vi "Swerve Module (Metric).vi"(0 "Y":dbl, 1 "X":dbl, 2 "Gyroscope":dbl, 3 "Rotation":dbl, 4 "alpha":dbl=50.64 format="%#_13g", 5 "error in":errorcluster, 7 "Steering Motor type":i32(ring) items=["Talon FX", "SPARK MAX", "Talon SRX"], 9 "Drive Motor type":i32(ring) items=["Talon FX", "SPARK MAX", "Talon SRX"], 11 "ticks per rev":dbl=2048.0 format="%#_13g", 13 "Gear Ratio":dbl=15.4286 format="%#_13g") -> (14 "Angle Out":dbl[](array[numeric]), 16 "Steering Postion Control":dbl[](array[numeric]), 18 "Drive Power":dbl[](array[numeric]), 19 "error out":errorcluster)   [LabVIEW 2020]
uses:
  <vilib>/Analysis/coordinate.llb/Angle Units.ctl
  <vilib>/Analysis/coordinate.llb/Angle Range (Degree).ctl
  <vilib>/Rock Robotics/WPI/ThirdParty/Phoenix-LabVIEW/Motor Controller/Controls/CTRE_Phoenix_MotorControl_TalonFXInvertType.ctl
  <vilib>/Analysis/coordinate.llb/Wrap Angle (scalar).vi
  <vilib>/Rock Robotics/WPI/ThirdParty/JAS_Junk/TrajLib/Conv_Deg_Radians.vi
  <vilib>/Rock Robotics/WPI/ThirdParty/JAS_Junk/TrajLib/Rotation2d_CreateAngle.vi
  <vilib>/Rock Robotics/WPI/ThirdParty/JAS_Junk/TrajLib/Util_CalcDist.vi
  <vilib>/Rock Robotics/WPI/ThirdParty/JAS_Junk/TrajLib/Rotation2d_UnaryMinus.vi
  <vilib>/Rock Robotics/WPI/Utilities/WPI_GetSetVariantRefNum.vi
  <vilib>/Rock Robotics/WPI/ThirdParty/Phoenix-LabVIEW/CANCoder/Get/CTRE_Phoenix_CANcoder_GetSensorData.vi
  <vilib>/Rock Robotics/WPI/ThirdParty/Phoenix-LabVIEW/Motor Controller/Get/CTRE_Phoenix_MotorController_GetSelectedSensorData.vi
  <vilib>/Rock Robotics/WPI/ThirdParty/JAS_Junk/TrajLib/Trajectory_Library.lvlib
  <vilib>/Analysis/NI_AAL_Angle.lvlib
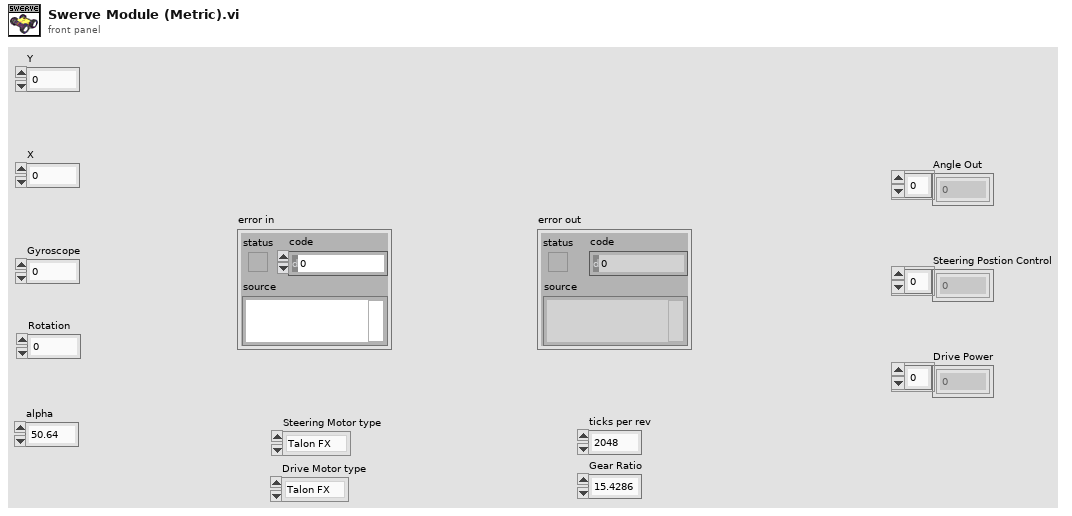
[diagram p1: front panel]
types:
  T1 = typedef "NI_AAL_Angle.lvlib/Angle Range (Degree).ctl" = u16
  T2 = typedef "NI_AAL_Angle.lvlib/Angle Units.ctl" = i32
  T3 = typedef "CTRE_Phoenix_CANcoder_DeviceRef.ctl" = cluster{"DeviceStatus":errorcluster, "Device Number":u8, "Handle":u64, "UsageFrame":u32, "Library Path":path}
  T4 = typedef "WPI_MotorControlDeviceRef.ctl" = cluster{"DeviceStatus":errorcluster, "Type":T5, "PWM":cluster{"PWM Channel":T6, "DeadBand":T7}, "CAN":cluster{"Device Number":u8, "SetOutput VI Ref":variant, "GetOutput VI Ref":variant, "Enable VI Ref":variant, "Disable VI Ref":variant, "Data":variant}, "Invert":bool, "DIO PWM":cluster{"PWM \"Enable\" Channel":T6, "DIOChannel":T8, "PWM Rate":dbl}}
  T5 = typedef "WPI_MotorControlType.ctl" = enum16{"PWM", "CAN", "DIO PWM"}
  T6 = typedef "FPGA_DIOPWMChannel.ctl" = enum8{"PWM 0", "PWM 1", "PWM 2", "PWM 3", "PWM 4", "PWM 5", "PWM 6", "PWM 7", "PWM 8", "PWM 9", "PWM MXP 0", "PWM MXP 1", "PWM MXP 2", "PWM MXP 3", "PWM MXP 4", "PWM MXP 5", "PWM MXP 6", "PWM MXP 7", "PWM MXP 8", "PWM MXP 9", "Invalid"}
  T7 = typedef "WPI_PWMDeadband.ctl" = cluster{"Name":string, "maxPositivePwm":i32, "minPositivePwm":i32, "centerPwm":i32, "maxNegativePwm":i32, "minNegativePwm":i32, "angularRange":u16}
  T8 = typedef "FPGA_DIOChannel.ctl" = enum8{"DIO 0", "DIO 1", "DIO 2", "DIO 3", "DIO 4", "DIO 5", "DIO 6", "DIO 7", "DIO 8", "DIO 9", "DIO MXP 0", "DIO MXP 1", "DIO MXP 2", "DIO MXP 3", "DIO MXP 4", "DIO MXP 5", "DIO MXP 6", "DIO MXP 7", "DIO MXP 8", "DIO MXP 9", "DIO MXP 10", "DIO MXP 11", "DIO MXP 12", "DIO MXP 13", "DIO MXP 14", "DIO MXP 15", "SPI Port CS1", "SPI Port CS2", "SPI Port CS3", "SPI Port MISO", "SPI Port MOSI", "Invalid"}
  T9 = typedef "Trajectory_Library.lvlib/ROTATION2D.ctl" = cluster{"VALUE":dbl, "COS":dbl, "SIN":dbl}
  T10 = typedef "WPI_JoystickDevRef.ctl" = cluster{"Device":T11}
  T11 = typedef "WPI_JoystickDeviceEnum.ctl" = enum16{"USB 0", "USB 1", "USB 2", "USB 3", "USB 4", "USB 5"}
  T12 = typedef "CTRE_Phoenix_MotorControl_TalonFXInvertType.ctl" = enum16{"Counter-Clockwise", "Clockwise"}
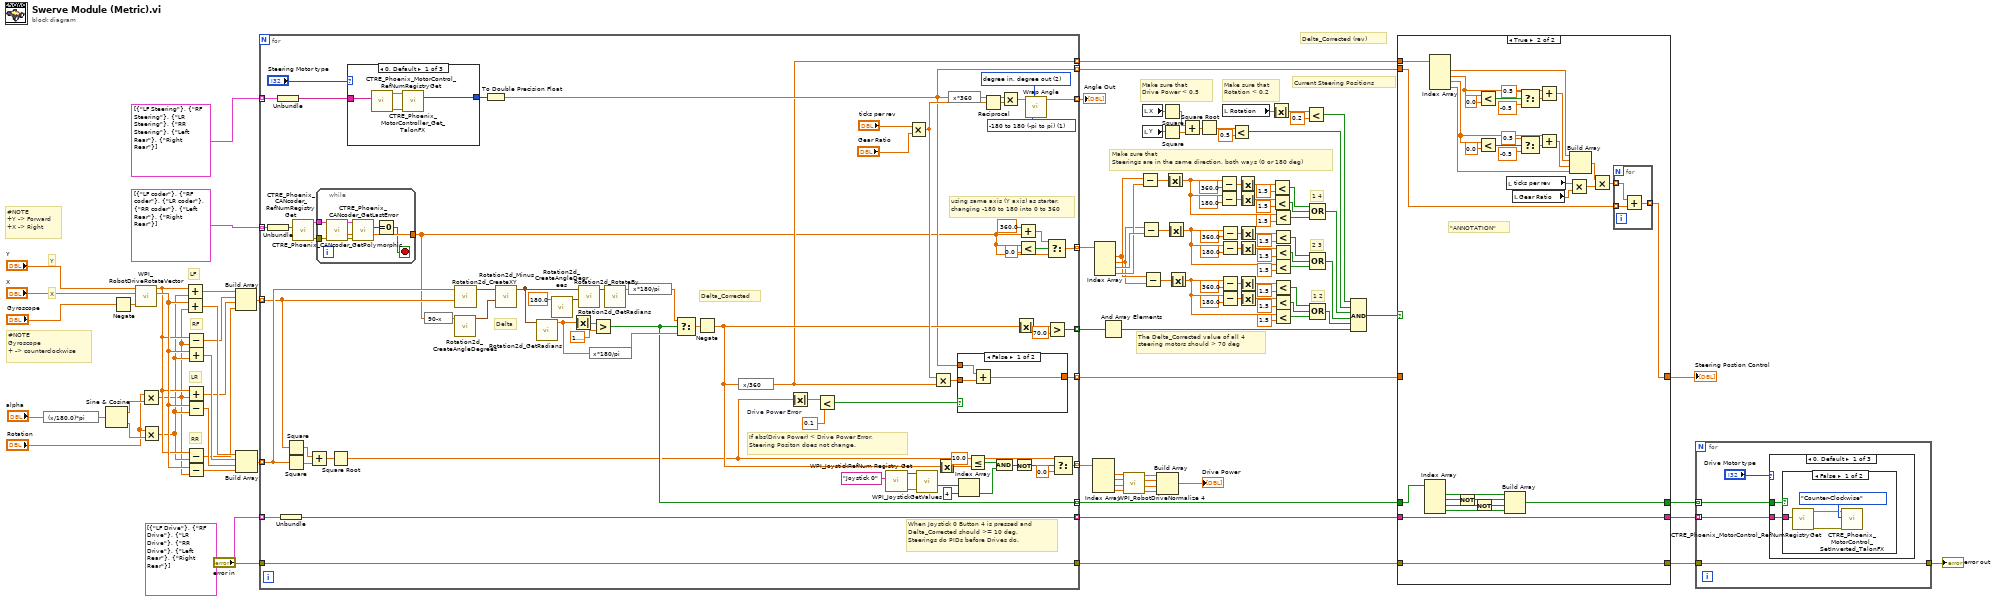
[diagram p0: block diagram]
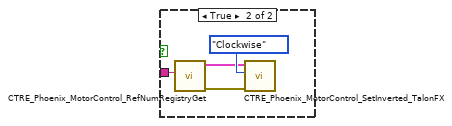
[diagram p3: hidden frame]
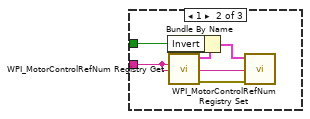
[diagram p4: hidden frame]
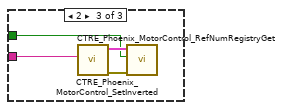
[diagram p5: hidden frame]
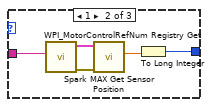
[diagram p6: hidden frame]
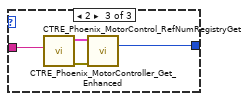
[diagram p7: hidden frame]
diagram:
  # "#NOTE\nGyroscope\n+ -> counterclockwise"
  # "#NOTE\n+Y -> Forward\n+X -> Right"
  # "Current Steering Positions"
  # "Delta_Corrected (rev)"
  # "Make sure that\nRotation < 0.2"
  # "Make sure that\nDrive Power < 0.5"
  # "The Delta_Corrected value of all 4 steering motors should > 70 deg"
  # "Make sure that\nSteerings are in the same direction, both ways (0 or 180 deg)"
  # "1 4"
  # "1 2"
  # "2 3"
  # "RR"
  # "LR"
  # "RF"
  # "LF"
  # "X"
  # "Y"
  n1 = expression code="(x/180.0)*pi" ("degrees to radians")("alpha") -> (w83:dbl)
  n2 = Sine & Cosine(0:w83) -> (1:w85:dbl, 2:w84:dbl)
  n3 = Negate(x="Gyroscope") -> (-x=w2:dbl)
  n4 = call <vilib>:"WPI_RobotDriveRotateVector.vi"("Angle"=w2, "X"="X", "Y"="Y") -> ("X'"=w90:dbl, "Y'"=w89:dbl)  [unwired: 7 out]
  n5 = Multiply(x="Rotation", y=w85) -> (x*y=w87:dbl)
  n6 = Multiply(x="Rotation", y=w84) -> (x*y=w88:dbl)
  n7 = Add(x=w89, y=w88) -> (x+y=w92:dbl)
  n8 = Add(x=w90, y=w87) -> (x+y=w96:dbl)
  n9 = Subtract(x=w89, y=w87) -> (x-y=w93:dbl)
  n10 = Add(x=w90, y=w88) -> (x+y=w97:dbl)
  n11 = Add(x=w89, y=w87) -> (x+y=w94:dbl)
  n12 = Subtract(x=w90, y=w88) -> (x-y=w98:dbl)
  n13 = Subtract(x=w89, y=w88) -> (x-y=w95:dbl)
  n14 = Subtract(x=w90, y=w87) -> (x-y=w99:dbl)
  n15 = Build Array(w92, w93, w94, w95) -> (w100:dbl[])
  n16 = Build Array(w96, w97, w98, w99) -> (w101:dbl[])
  n17 = for {
    tunnel: w100 -> [w147] mode=indexing
    tunnel: w101 -> [w148] mode=indexing
    tunnel: [w129] -> w108 mode=indexing
    tunnel: cluster{string}[] [{"LF Steering"}, {"RF Steering"}, {"LR Steering"}, {"RR Steering"}, {"Left Rear"}, {"Right Rear"}] ("Steering ref") -> [w182] mode=indexing
    tunnel: cluster{string}[] [{"LF coder"}, {"RF coder"}, {"LR coder"}, {"RR coder"}, {"Left Rear"}, {"Right Rear"}] ("CANcoder ref") -> [w178] mode=indexing
    tunnel: cluster{string}[] [{"LF Drive"}, {"RF Drive"}, {"LR Drive"}, {"RR Drive"}, {"Left Rear"}, {"Right Rear"}] ("Drive ref") -> [w173] mode=indexing
    tunnel: [w172] -> w77 mode=indexing
    tunnel: [w133] -> w48 mode=indexing
    tunnel: "error in" -> [w163]
    tunnel: [w163] -> w75
    tunnel: [w146] -> w81 mode=indexing
    tunnel: [w145] -> w79 mode=indexing
    tunnel: [w142] -> w49 mode=indexing
    tunnel: [w137] -> w50 mode=indexing
    tunnel: [w117] -> w6 mode=indexing
    tunnel: [w116] -> w5 mode=indexing
    w136 = T1 1 items=["none", "-180 to 180 (-pi to pi)", "0 to 360 (0 to 2pi)"] ("angle range")
    w135 = T2 2 items=["radian in, radian out", "radian in, degree out", "degree in, degree out", "degree in, radian out"] ("angle units")
    w175 = 0.1  # Drive Power Error
    # "When Joystick 0 Button 4 is pressed and Delta_Corrected should >= 10 deg,\nSteerings do PIDs before Drives do."
    # "Delta_Corrected"
    # "using same axis (Y axis) as starter,\nchanging -180 to 180 into 0 to 360"
    # "If abs(Drive Power) < Drive Power Error,\nSteering Positon does not change."
    # "Delta"
    n18 = Unbundle(w178) -> (w177:string)
    n19 = Unbundle(w182) -> (w181:string)
    n20 = Unbundle(w173) -> (w146:string)
    n21 = Square(x=w147) -> (x^2=w183:dbl)
    n22 = Square(x=w148) -> (x^2=w184:dbl)
    n23 = call <vilib>:"CTRE_Phoenix_CANcoder_RefNumRegistryGet.vi"("refnum name"=w177) -> ("error out"=w180:errorcluster, "CTRE_CANcoder_DeviceRef"=w179:T3)  [unwired: 9 in]
    n24 = Add(x=w183, y=w184) -> (x+y=w185:dbl)
    n25 = while {
      tunnel: w180 -> [w192]
      tunnel: w179 -> [w191]
      tunnel: [w187] -> w115
      stop <- w186 stop-if-true
      n26 = call-poly <vilib>:"CTRE_Phoenix_CANcoder_GetPolymorphic.vi"("CTRE_CANcoder_DeviceRef"=w191, "error in"=w192) -> ("CTRE_CANcoder_DeviceRef"=w190:T3, "Absolute Position"=w187:dbl, "error out"=w189:errorcluster)  [unwired: 9 in, 2 out]
      n27 = call <vilib>:"CTRE_Phoenix_CANcoder_GetLastError.vi"("error in"=w189, "CTRE_CANcoder_DeviceRef"=w190) -> ("Last Error Code"=w188:i8)  [unwired: 7 in, 2 out]
      n28 = Equal To 0?(x=w188) -> (x = 0?=w186:bool)
    }
    n29 = Square Root(x=w185) -> (sqrt(x)=w130:dbl)
    n30 = case shown="0, Default" "Steering Motor type" {
      tunnel: w181 -> [w194 w201 w203]
      tunnel: [w193 w197 w202] -> w176
      frame 0, Default {
        n31 = call <vilib>:"CTRE_Phoenix_MotorControl_RefNumRegistryGet.vi"("refnum name"=w194) -> ("error out"=w196:errorcluster, "PhoenixMotorControlDevRef"=w195:T4)  [unwired: 9 in]
        n32 = call-poly <vilib>:"CTRE_Phoenix_MotorController_Get_TalonFX.vi"("PhoenixMotorControlDevRef"=w195, "error in"=w196) -> ("Position (Raw Sensor Units)"=w193:i32)  [unwired: 10 in, 3 out]
      }
      frame 1 {
        n33 = call <vilib>:"WPI_MotorControlRefNum Registry Get.vi"("refnum name"=w201) -> ("error out"=w200:errorcluster, "MotorControlDevRef"=w199:T4)  [unwired: 9 in]
        n34 = call <vilib>:"Spark MAX Get Sensor Position.vi"("error in (no error)"=w200, "MotorControlDevRef in"=w199) -> ("Sensor Position"=w198:dbl)  [unwired: 6 in, 3 out]
        n35 = To Long Integer(number=w198) -> (32bit integer=w197:i32)
      }
      frame 2 {
        n36 = call <vilib>:"CTRE_Phoenix_MotorControl_RefNumRegistryGet.vi"("refnum name"=w203) -> ("error out"=w204:errorcluster, "PhoenixMotorControlDevRef"=w205:T4)  [unwired: 9 in]
        n37 = call-poly <vilib>:"CTRE_Phoenix_MotorController_Get_Enhanced.vi"("PhoenixMotorControlDevRef"=w205, "error in"=w204) -> ("Position (Raw Sensor Units)"=w202:i32)  [unwired: 10 in, 3 out]
      }
    }
    n38 = expression code="90-x"(w115) -> (w160:dbl)
    n39 = call <vilib>:"Rotation2d_CreateAngleDegrees.vi"("Angle_Degrees"=w160) -> ("ROTATION"=w159:T9)  [unwired: 10 in]
    n40 = call <vilib>:"Rotation2d_CreateXY.vi"("Y or sine"=w147, "X or  cosine"=w148) -> ("ROTATION"=w158:T9)  [unwired: 9 in]
    n41 = To Double Precision Float(number=w176) -> (double precision float=w117:dbl)
    n42 = call <vilib>:"Rotation2d_Minus.vi"("other ROTATION"=w159, "in ROTATION"=w158) -> ("out ROTATION"=w154:T9)  [unwired: 9 in]
    n43 = call <vilib>:"Rotation2d_GetRadians.vi"("in ROTATION"=w154) -> ("AngleRadians"=w157:dbl)  [unwired: 10 in]
    n44 = call <vilib>:"Rotation2d_CreateAngleDegrees.vi"("Angle_Degrees"=180.0) -> ("ROTATION"=w156:T9)  [unwired: 10 in]
    n45 = Absolute Value(x=w157) -> (abs(x)=w161:dbl)
    n46 = call <vilib>:"Rotation2d_RotateBy.vi"("other Rotation"=w156, "in ROTATION"=w154) -> ("out ROTATION"=w153:T9)  [unwired: 9 in]
    n47 = expression code="x*180/pi"(w157) -> (w150:dbl)
    n48 = Greater?(x=w161, y=1.5707963267948966) -> (0:w145:bool)
    n49 = call <vilib>:"Rotation2d_GetRadians.vi"("in ROTATION"=w153) -> ("AngleRadians"=w152:dbl)  [unwired: 10 in]
    n50 = expression code="x*180/pi"(w152) -> (w151:dbl)
    n51 = Select(t=w151, s=w145, f=w150) -> (s? t:f=w149:dbl)
    n52 = Negate(x=w149) -> (-x=w132:dbl)
    n53 = expression code="x/360"(w132) -> (w116:dbl)
    n54 = Absolute Value(x=w130) -> (abs(x)=w174:dbl)
    n55 = Less?(x=w174, y=w175) -> (x < y?=w171:bool)
    n56 = call <vilib>:"WPI_JoystickRefNum Registry Get.vi"("refnum name"="Joystick 0") -> ("error out"=w122:errorcluster, "JoystickDevRef"=w123:T10)  [unwired: 1 in, 8 out]
    n57 = Multiply(x="ticks per rev", y="Gear Ratio") -> (x*y=w164:dbl)
    n58 = call <vilib>:"WPI_JoystickGetValues.vi"("error in (no error)"=w122, "JoystickDevRef"=w123) -> ("Buttons"=w124:bool[])  [unwired: 5 in, 4 out]
    n59 = Multiply(x=w164, y=w116) -> (x*y=w165:dbl)
    n60 = Absolute Value(x=w132) -> (abs(x)=w126:dbl)
    n61 = expression code="x*360"(w117) -> (w166:dbl)
    n62 = case shown="False" w171 {
      tunnel: w165 -> [w208 _]
      tunnel: [w207 w209] -> w172
      tunnel: w117 -> [w206 w209]
      frame False {
        n63 = Add(x=w206, y=w208) -> (x+y=w207:dbl)
      }
      frame True {
      }
    }
    n64 = Index Array(array=w124, index=4) -> (element=w119:bool)
    n65 = Less Or Equal?(x=10.0, y=w126) -> (x <= y?=w131:bool)
    n66 = Reciprocal(x=w164) -> (1/x=w167:dbl)
    n67 = And(x=w131, y=w119) -> (x .and. y?=w128:bool)
    n68 = Multiply(x=w166, y=w167) -> (x*y=w134:dbl)
    n69 = Not(x=w128) -> (.not. x?=w127:bool)
    n70 = Absolute Value(x=w132) -> (abs(x)=w144:dbl)
    n71 = Add(x=360.0, y=w115) -> (x+y=w140:dbl)
    n72 = Less?(x=w115, y=0.0) -> (x < y?=w139:bool)
    n73 = call-poly <vilib>:"Wrap Angle.vi"("angle units"=w135, "angle range"=w136, "angle in"=w134) -> ("angle out"=w133:dbl)  [unwired: 7 in, 1 out]
    n74 = Select(t=w140, s=w139, f=w115) -> (s? t:f=w137:dbl)
    n75 = Greater?(x=w144, y=70.0) -> (0:w142:bool)
    n76 = Select(t=w130, s=w127, f=0.0) -> (s? t:f=w129:dbl)
  }
  "Angle Out" <- w48
  n77 = Index Array(array=w108) -> (element #1=w102:dbl, element #2=w103:dbl, element #3=w104:dbl, element #4=w105:dbl)  [unwired: 4 in]
  n78 = Index Array(array=w50) -> (element #1=w65:dbl, element #2=w64:dbl, element #3=w72:dbl, element #4=w69:dbl)  [unwired: 4 in]
  n79 = And Array Elements(Boolean array=w49) -> (logical AND=w23:bool)
  n80 = call <vilib>:"WPI_RobotDriveNormalize 4.vi"("D"=w105, "C"=w104, "B"=w103, "A"=w102) -> ("D'"=w111:dbl, "C'"=w112:dbl, "B'"=w113:dbl, "A'"=w114:dbl)
  n81 = Subtract(x=w65, y=w69) -> (x-y=w71:dbl)
  n82 = Subtract(x=w64, y=w72) -> (x-y=w70:dbl)
  n83 = local read "X"() -> (w18:dbl)
  n84 = local read "Y"() -> (w17:dbl)
  n85 = Subtract(x=w65, y=w64) -> (x-y=w66:dbl)
  n86 = Build Array(w114, w113, w112, w111) -> (→"Drive Power":dbl[])
  n87 = Square(x=w18) -> (x^2=w16:dbl)
  n88 = Square(x=w17) -> (x^2=w15:dbl)
  n89 = Absolute Value(x=w71) -> (abs(x)=w38:dbl)
  n90 = Absolute Value(x=w70) -> (abs(x)=w43:dbl)
  n91 = Absolute Value(x=w66) -> (abs(x)=w33:dbl)
  n92 = Add(x=w16, y=w15) -> (x+y=w14:dbl)
  n93 = Square Root(x=w14) -> (sqrt(x)=w9:dbl)
  n94 = Subtract(x=w38, y=360.0) -> (x-y=w41:dbl)
  n95 = Subtract(x=w38, y=180.0) -> (x-y=w52:dbl)
  n96 = Subtract(x=w43, y=360.0) -> (x-y=w45:dbl)
  n97 = Subtract(x=w43, y=180.0) -> (x-y=w57:dbl)
  n98 = Subtract(x=w33, y=360.0) -> (x-y=w36:dbl)
  n99 = Subtract(x=w33, y=180.0) -> (x-y=w62:dbl)
  n100 = local read "Rotation"() -> (w11:dbl)
  n101 = Less?(x=w9, y=0.5) -> (x < y?=w8:bool)
  n102 = Absolute Value(x=w41) -> (abs(x)=w40:dbl)
  n103 = Absolute Value(x=w52) -> (abs(x)=w51:dbl)
  n104 = Absolute Value(x=w45) -> (abs(x)=w44:dbl)
  n105 = Absolute Value(x=w57) -> (abs(x)=w56:dbl)
  n106 = Absolute Value(x=w36) -> (abs(x)=w35:dbl)
  n107 = Absolute Value(x=w62) -> (abs(x)=w61:dbl)
  n108 = Absolute Value(x=w11) -> (abs(x)=w13:dbl)
  n109 = Less?(x=w40, y=1.5) -> (x < y?=w24:bool)
  n110 = Less?(x=w51, y=1.5) -> (x < y?=w25:bool)
  n111 = Less?(x=w38, y=1.5) -> (x < y?=w26:bool)
  n112 = Less?(x=w44, y=1.5) -> (x < y?=w27:bool)
  n113 = Less?(x=w56, y=1.5) -> (x < y?=w28:bool)
  n114 = Less?(x=w35, y=1.5) -> (x < y?=w30:bool)
  n115 = Less?(x=w61, y=1.5) -> (x < y?=w31:bool)
  n116 = Less?(x=w43, y=1.5) -> (x < y?=w29:bool)
  n117 = Less?(x=w33, y=1.5) -> (x < y?=w32:bool)
  n118 = Less?(x=w13, y=0.2) -> (x < y?=w7:bool)
  n119 = Compound Arithmetic op=OR(w24, w25, w26) -> (w20:bool)
  n120 = Compound Arithmetic op=OR(w27, w28, w29) -> (w21:bool)
  n121 = Compound Arithmetic op=OR(w30, w31, w32) -> (w22:bool)
  n122 = Compound Arithmetic op=AND(w7, w8, w20, w21, w22, w23) -> (w19:bool)
  n123 = case shown="True" w19 {
    tunnel: w81 -> [w212 w247]
    tunnel: [w212 w247] -> w80
    tunnel: w79 -> [w213 w240]
    tunnel: [w213 w238] -> w78
    tunnel: w77 -> [w211 _]
    tunnel: [w211 w214] -> w76
    tunnel: w75 -> [w210 w246]
    tunnel: [w210 w246] -> w74
    tunnel: w6 -> [_ w216]
    tunnel: w5 -> [_ w221]
    frame False {
    }
    frame True {
      # "\"ANNOTATION\""
      n124 = Index Array(array=w240) -> (element #1=w239:bool, element #2=w244:bool, element #3=w241:bool, element #4=w245:bool)  [unwired: 4 in]
      n125 = Index Array(array=w221) -> (element #1=w227:dbl, element #2=w228:dbl, element #3=w222:dbl, element #4=w224:dbl)  [unwired: 4 in]
      n126 = Not(x=w244) -> (.not. x?=w243:bool)
      n127 = Not(x=w241) -> (.not. x?=w242:bool)
      n128 = Less?(x=w228, y=0.0) -> (x < y?=w235:bool)
      n129 = Less?(x=w222, y=0.0) -> (x < y?=w230:bool)
      n130 = Build Array(w239, w243, w242, w245) -> (w238:bool[])
      n131 = local read "ticks per rev"() -> (w219:dbl)
      n132 = local read "Gear Ratio"() -> (w220:dbl)
      n133 = Select(t=0.5, s=w235, f=-0.5) -> (s? t:f=w229:dbl)
      n134 = Select(t=0.5, s=w230, f=-0.5) -> (s? t:f=w223:dbl)
      n135 = Add(x=w228, y=w229) -> (x+y=w226:dbl)
      n136 = Add(x=w222, y=w223) -> (x+y=w225:dbl)
      n137 = Multiply(x=w219, y=w220) -> (x*y=w218:dbl)
      n138 = Build Array(w227, w226, w225, w224) -> (w217:dbl[])
      n139 = Multiply(x=w217, y=w218) -> (x*y=w215:dbl[])
      n140 = for {
        tunnel: [w250] -> w214 mode=indexing
        tunnel: w216 -> [w249] mode=indexing
        tunnel: w215 -> [w248] mode=indexing
        n141 = Add(x=w248, y=w249) -> (x+y=w250:dbl)
      }
    }
  }
  "Steering Postion Control" <- w76
  n142 = for {
    tunnel: w80 -> [w253] mode=indexing
    tunnel: w78 -> [w252] mode=indexing
    tunnel: w74 -> [w251]
    tunnel: [w251] -> w73
    n143 = case shown="0, Default" "Drive Motor type" {
      tunnel: w253 -> [w256 w268 w273]
      tunnel: w252 -> [w255 w266 w270]
      frame 0, Default {
        n144 = case shown="False" w255 {
          tunnel: w256 -> [w259 w263]
          frame False {
            n145 = call <vilib>:"CTRE_Phoenix_MotorControl_RefNumRegistryGet.vi"("refnum name"=w259) -> ("error out"=w257:errorcluster, "PhoenixMotorControlDevRef"=w258:T4)  [unwired: 9 in]
            n146 = call <vilib>:"CTRE_Phoenix_MotorControl_SetInverted_TalonFX.vi"("error in (no error)"=w257, "Invert Type"=CTRE_Phoenix_MotorControl_TalonFXInvertType."Counter-Clockwise", "PhoenixMotorControlDevRef"=w258) -> ()  [unwired: 7 in, 2 out]
          }
          frame True {
            n147 = call <vilib>:"CTRE_Phoenix_MotorControl_RefNumRegistryGet.vi"("refnum name"=w263) -> ("error out"=w261:errorcluster, "PhoenixMotorControlDevRef"=w262:T4)  [unwired: 9 in]
            n148 = call <vilib>:"CTRE_Phoenix_MotorControl_SetInverted_TalonFX.vi"("error in (no error)"=w261, "Invert Type"=CTRE_Phoenix_MotorControl_TalonFXInvertType."Clockwise", "PhoenixMotorControlDevRef"=w262) -> ()  [unwired: 7 in, 2 out]
          }
        }
      }
      frame 1 {
        n149 = call <vilib>:"WPI_MotorControlRefNum Registry Get.vi"("refnum name"=w268) -> ("error out"=w265:errorcluster, "MotorControlDevRef"=w267:T4)  [unwired: 9 in]
        n150 = Bundle By Name(cluster=w267, "Invert"=w266) -> (w269:T4)
        n151 = call <vilib>:"WPI_MotorControlRefNum Registry Set.vi"("error in (no error)"=w265, "refnum name"=w268, "MotorControlDevRef"=w269) -> ()  [unwired: 7 in, 2 out]
      }
      frame 2 {
        n152 = call <vilib>:"CTRE_Phoenix_MotorControl_RefNumRegistryGet.vi"("refnum name"=w273) -> ("error out"=w272:errorcluster, "PhoenixMotorControlDevRef"=w271:T4)  [unwired: 9 in]
        n153 = call <vilib>:"CTRE_Phoenix_MotorControl_SetInverted.vi"("error in (no error)"=w272, "Invert?"=w270, "PhoenixMotorControlDevRef"=w271) -> ()  [unwired: 7 in, 2 out]
      }
    }
  }
  "error out" <- w73
